vi "Calculate Pulse Current.vi"(10 "Load Resistance":dbl=400.0, 11 "Waveform Array":waveform(dbl)[](array[waveform])) -> (0 "error out":errorcluster, 3 "Pulse Currents":dbl[](array[numeric]))   [LabVIEW 2010]
uses:
  <vilib>/measure/mamon.llb/Trigger Detection for 1 Channel.vi
  <vilib>/measure/NI_MAPro.lvlib
  <vilib>/Analysis/NI_AALBase.lvlib
panel:
  out "Waveform Array 2":waveform(dbl)[](graph)
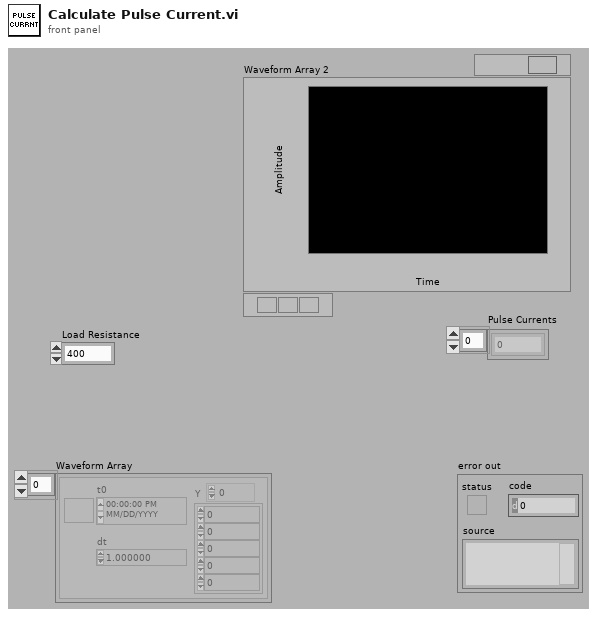
[diagram p1: front panel]
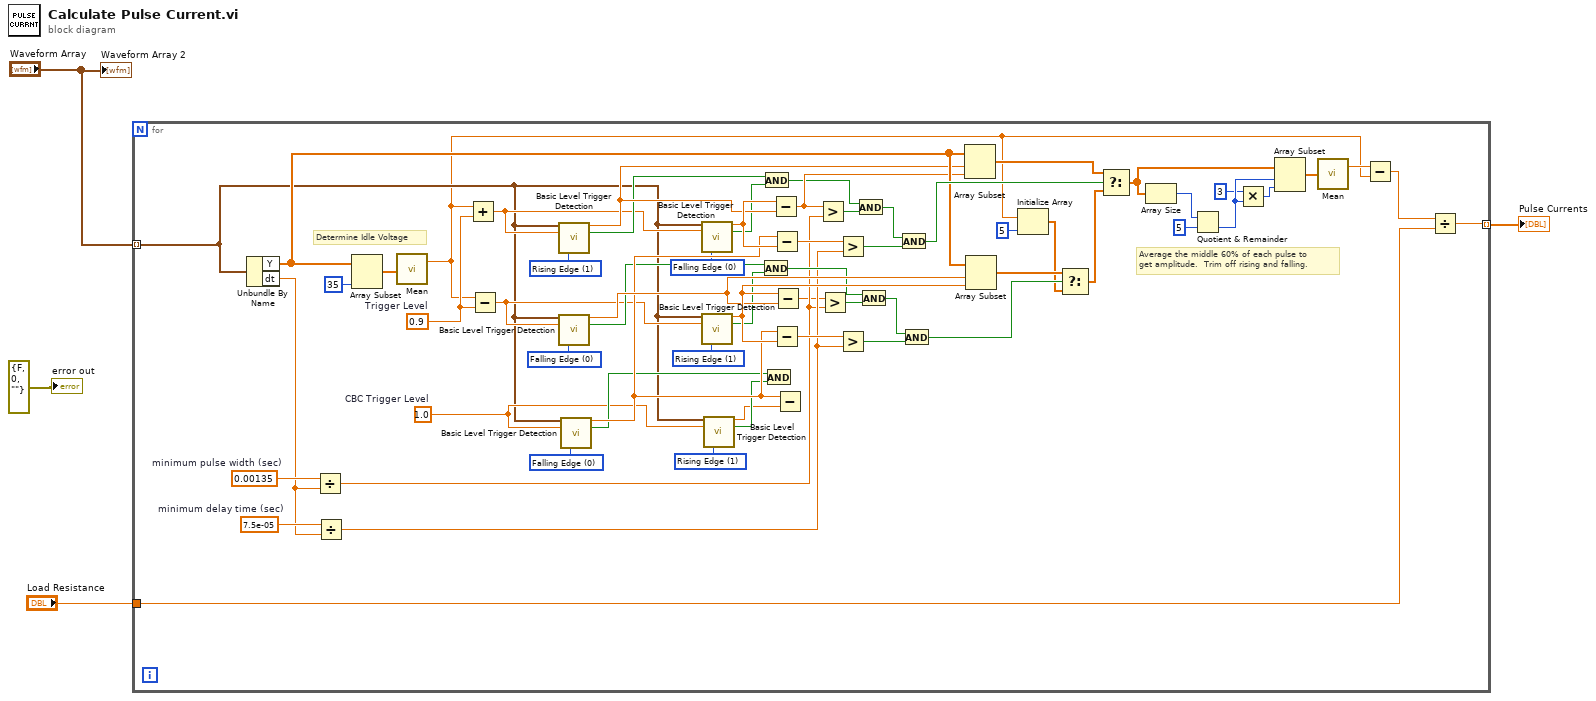
[diagram p0: block diagram]
diagram:
  n1 = for {
    tunnel: "Waveform Array" -> [w13] mode=indexing
    tunnel: [w9] -> w4 mode=indexing
    tunnel: "Load Resistance" -> [w10]
    w39 = 7.5e-05  # minimum delay time (sec)
    w33 = 0.00135  # minimum pulse width (sec)
    w26 = 1.0  # CBC Trigger Level
    w24 = u16 1 items=["Falling Edge", "Rising Edge"] ("trigger slope")
    w23 = u16 0 items=["Falling Edge", "Rising Edge"] ("trigger slope")
    w20 = u16 1 items=["Falling Edge", "Rising Edge"] ("trigger slope")
    w19 = u16 0 items=["Falling Edge", "Rising Edge"] ("trigger slope")
    w18 = 0.9  # Trigger Level
    w17 = u16 0 items=["Falling Edge", "Rising Edge"] ("trigger slope")
    w14 = u16 1 items=["Falling Edge", "Rising Edge"] ("trigger slope")
    # "Average the middle 60% of each pulse to\nget amplitude.  Trim off rising and falling."
    # "Determine Idle Voltage"
    n2 = Unbundle By Name(w13) -> ("Y"=w54:dbl[], "dt"=w12:dbl)
    n3 = Divide(x=w33, y=w12) -> (x/y=w35:dbl)
    n4 = Divide(x=w39, y=w12) -> (x/y=w40:dbl)
    n5 = Array Subset(array=w54, length=35) -> (w16:dbl[])  [unwired: 1 in]
    n6 = call <vilib>:"Mean.vi"("X"=w16) -> ("mean"=w6:dbl)  [unwired: 1 out]
    n7 = Add(x=w6, y=w18) -> (x+y=w21:dbl)
    n8 = Subtract(x=w6, y=w18) -> (x-y=w22:dbl)
    n9 = call-poly <vilib>:"Basic Level Trigger Detection.vi"("signal in"=w13, "level"=w21, "trigger slope"=w14) -> ("trigger location"=w49:dbl, "trigger detected?"=w27:bool)  [unwired: 10 in, 1 out]
    n10 = call-poly <vilib>:"Basic Level Trigger Detection.vi"("signal in"=w13, "level"=w22, "trigger slope"=w17) -> ("trigger location"=w52:dbl, "trigger detected?"=w29:bool)  [unwired: 10 in, 1 out]
    n11 = call-poly <vilib>:"Basic Level Trigger Detection.vi"("signal in"=w13, "level"=w26, "trigger slope"=w23) -> ("trigger location"=w38:dbl, "trigger detected?"=w31:bool)  [unwired: 10 in, 1 out]
    n12 = call-poly <vilib>:"Basic Level Trigger Detection.vi"("signal in"=w13, "level"=w21, "trigger slope"=w19) -> ("trigger location"=w50:dbl, "trigger detected?"=w28:bool)  [unwired: 10 in, 1 out]
    n13 = call-poly <vilib>:"Basic Level Trigger Detection.vi"("signal in"=w13, "level"=w22, "trigger slope"=w20) -> ("trigger location"=w53:dbl, "trigger detected?"=w30:bool)  [unwired: 10 in, 1 out]
    n14 = call-poly <vilib>:"Basic Level Trigger Detection.vi"("signal in"=w13, "level"=w26, "trigger slope"=w24) -> ("trigger location"=w25:dbl, "trigger detected?"=w32:bool)  [unwired: 10 in, 1 out]
    n15 = And(x=w29, y=w30) -> (x .and. y?=w45:bool)
    n16 = And(x=w27, y=w28) -> (x .and. y?=w37:bool)
    n17 = And(x=w31, y=w32) -> ()  [unwired: 1 out]
    n18 = Subtract(x=w50, y=w49) -> (x-y=w51:dbl)
    n19 = Subtract(x=w38, y=w50) -> (x-y=w41:dbl)
    n20 = Subtract(x=w38, y=w53) -> (x-y=w42:dbl)
    n21 = Subtract(x=w53, y=w52) -> (x-y=w34:dbl)
    n22 = Subtract(x=w38, y=w25) -> ()  [unwired: 1 out]
    n23 = Greater?(x=w51, y=w35) -> (0:w36:bool)
    n24 = Greater?(x=w34, y=w35) -> (0:w46:bool)
    n25 = Greater?(x=w41, y=w40) -> (0:w44:bool)
    n26 = Greater?(x=w42, y=w40) -> (0:w48:bool)
    n27 = And(x=w37, y=w36) -> (x .and. y?=w43:bool)
    n28 = And(x=w45, y=w46) -> (x .and. y?=w47:bool)
    n29 = And(x=w43, y=w44) -> (x .and. y?=w56:bool)
    n30 = And(x=w47, y=w48) -> (x .and. y?=w58:bool)
    n31 = Array Subset(array=w54, index=w49, length=w51) -> (w55:dbl[])
    n32 = Array Subset(array=w54, index=w52, length=w53) -> (w57:dbl[])
    n33 = Initialize Array(w6, 5 ("dimension size")) -> (w5:dbl[])
    n34 = Select(t=w57, s=w58, f=w5) -> (s? t:f=w59:dbl[])
    n35 = Select(t=w55, s=w56, f=w59) -> (s? t:f=w66:dbl[])
    n36 = Array Size(array=w66) -> (size(s)=w60:i32)
    n37 = Quotient & Remainder(x=w60, y=5) -> (floor(x/y)=w63:i32)  [unwired: 1 out]
    n38 = Multiply(x=3, y=w63) -> (x*y=w64:i32)
    n39 = Array Subset(array=w66, index=w63, length=w64) -> (w65:dbl[])
    n40 = call <vilib>:"Mean.vi"("X"=w65) -> ("mean"=w11:dbl)  [unwired: 1 out]
    n41 = Subtract(x=w11, y=w6) -> (x-y=w8:dbl)
    n42 = Divide(x=w8, y=w10) -> (x/y=w9:dbl)
  }
  "Pulse Currents" <- w4
  "error out" <- errorcluster {"status"=FALSE, "code"=0, "source"=""} ("error out")
  "Waveform Array 2" <- "Waveform Array"
